vi "m1m3_getEvent_HardpointActuatorMotionState.vi"(8 "error in (no error)":errorcluster, 11 "logevent_HardpointActuatorMotionState_Ctl":T1={"Timestamp"=0.0, "MotionState[6]"=[0, 0, 0, 0, 0, 0], "priority"=0}) -> (0 "error out":errorcluster, 2 "function return":i32, 3 "logevent_HardpointActuatorMotionState_Ctl out":T1)   [LabVIEW 2016, in "SALLV_m1m3.lvlib"]
doc: "int m1m3_shm_getEvent_HardpointActuatorMotionStateLV(m1m3_logevent_HardpointActuatorMotionStateLV *logevent_HardpointActuatorMotionState_Ctl );"
uses:
  SALLV_m1m3.lvlib
  DataTypes/logevent_HardpointActuatorMotionState.ctl
  SALLV_m1m3.so
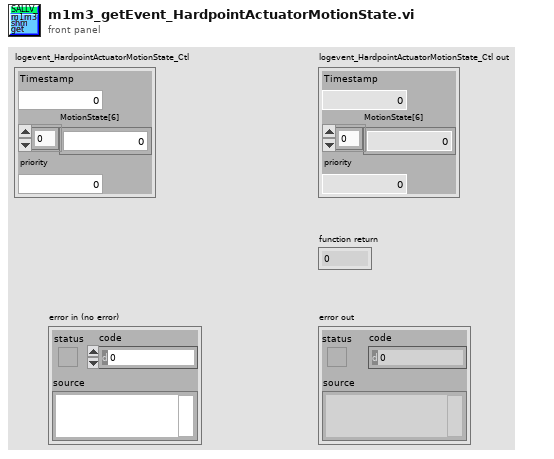
[diagram p1: front panel]
types:
  T1 = typedef "SALLV_m1m3.lvlib/logevent_HardpointActuatorMotionState.ctl" = cluster{"Timestamp":dbl, "MotionState[6]":i32[], "priority":i32}
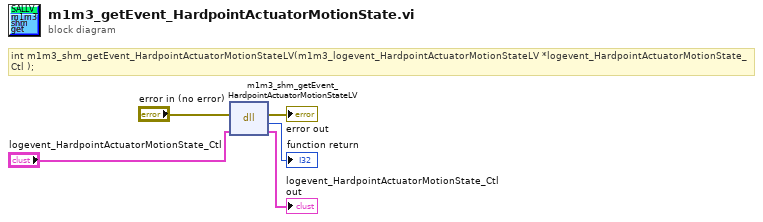
[diagram p0: block diagram]
diagram:
  # "int m1m3_shm_getEvent_HardpointActuatorMotionStateLV(m1m3_logevent_HardpointActuatorMotionStateLV *logevent_HardpointActuatorMotionState_Ctl );"
  n1 = dll-call lib="opt/CODE/ts_m1m3supporteui/SALLV_m1m3/SALLV_m1m3.*" fn="m1m3_shm_getEvent_HardpointActuatorMotionStateLV"(error in="error in (no error)", "logevent_HardpointActuatorMotionState_Ctl"="logevent_HardpointActuatorMotionState_Ctl") -> (error out=→"error out":errorcluster, →"function return":i32, "logevent_HardpointActuatorMotionState_Ctl"=→"logevent_HardpointActuatorMotionState_Ctl out":T1)  [unwired: 2 in, 1 out]
